vi "E_where_equal_to_dec.vi"(4 "Input array":i32[](array[numeric]), 5 "y":i16) -> (0 "String":string, 1 "Index array":i32[](array[numeric]), 2 "Incrimentor":i32)   [LabVIEW 2013]
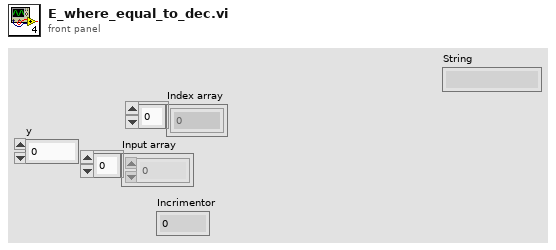
[diagram p1: front panel]
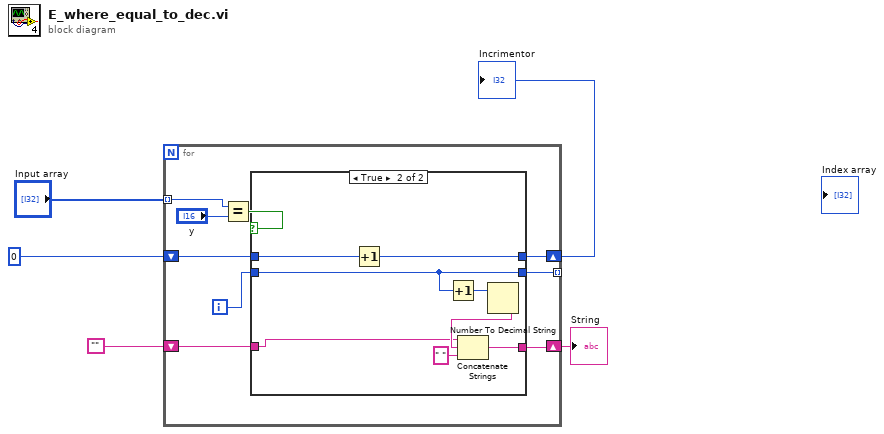
[diagram p0: block diagram]
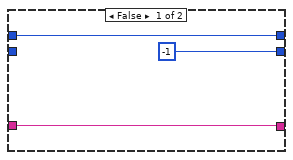
[diagram p2: hidden frame]
diagram:
  n1 = for {
    tunnel: "Input array" -> [w14] mode=indexing
    tunnel: [w11] -> _ mode=indexing
    shift-right: [w8] -> w3
    shift-left: 0 -> [w9]
    shift-right: [w6] -> w1
    shift-left: "" -> [w7]
    i -> [w12]
    n2 = Equal?(x=w14, y="y") -> (x = y?=w13:bool)
    n3 = case shown="True" w13 {
      tunnel: w12 -> [_ w20]
      tunnel: [-1 w20] -> w11
      tunnel: w9 -> [w16 w25]
      tunnel: [w16 w24] -> w8
      tunnel: w7 -> [w15 w18]
      tunnel: [w15 w21] -> w6
      frame False {
      }
      frame True {
        n4 = Increment(x=w25) -> (x+1=w24:i32)
        n5 = Increment(x=w20) -> (x+1=w19:i32)
        n6 = Number To Decimal String(number=w19) -> (decimal integer string=w23:string)  [unwired: 1 in]
        n7 = Concatenate Strings(w18, w23, " " ("string")) -> (w21:string)
      }
    }
  }
  "Incrimentor" <- w3
  "String" <- w1
